vi "Do Request.vi"(7 "Processing In":refnum<class "Processing.lvclass">, 11 "TemplatedFileServe in":refnum<class "TemplatedFileServe.lvclass">) -> (0 "error out":errorcluster, 5 "Processing":refnum<class "Processing.lvclass">)   [LabVIEW 2020, in "HTTP Server.lvlib" / "TemplatedFileServe.lvclass"]
doc: "A controller's main job is to respond to a request by generating a response. The response value must be specified by calling Set Response.vi on the Processing class that's passed through the VI otherwise an error will be generated.\n\nThere are several helpers available for common response types:\nGenerating HTML content programmatically - Create Basic Response.vi\nStreaming a file from disk - Create File Response.vi\nRedirecting the user to another URL - Create Redirect Response.vi\n\nFile responses are streamed in chunks and do not load the entire file into memory at once to send in the response which allows serving large files more efficiently."
uses:
  TemplatedFileServe.lvclass
  Processing/Processing.lvclass
  Processing/Processing.lvclass/Processing.ctl
  lv-http-util/HTTP Utils/Request/Request.lvclass/Request.ctl
  lv-uri/URI/URI/URI.lvclass/URI.ctl
  TemplatedFileServe.lvclass/TemplatedFileServe.ctl
  StandardFileServe/StandardFileServe.lvclass
  lv-http-util/HTTP Utils/Request/Request.lvclass
  lv-uri/URI/URI/URI.lvclass
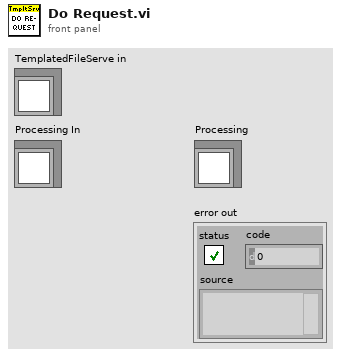
[diagram p1: front panel]
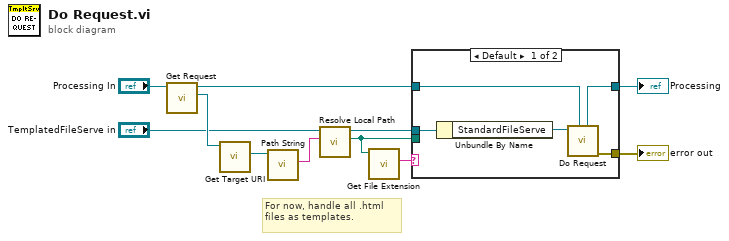
[diagram p0: block diagram]
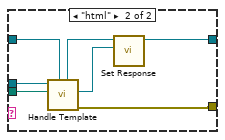
[diagram p2: hidden frame]
diagram:
  # "For now, handle all .html files as templates."
  n1 = call "Get Request.vi"("Processing in"="Processing In") -> ("Request"=w10:refnum<class "Request.lvclass">, "Processing out"=w4:refnum<class "Processing.lvclass">)  [unwired: 9 in]
  n2 = call "Get Target URI.vi"("Request in"=w10) -> ("Target URI"=w11:refnum<class "URI.lvclass">)  [unwired: 8 in, 2 out]
  n3 = call "Path String.vi"("URI in"=w11) -> ("Path String"=w7:string)  [unwired: 9 in, 1 out]
  n4 = call "Resolve Local Path.vi"("Request Path"=w7, "TemplatedFileServe in"="TemplatedFileServe in") -> ("Path"=w1:path, "TemplatedFileServe out"=w5:refnum<class "TemplatedFileServe.lvclass">)  [unwired: 7 in, 1 out]
  n5 = call <vilib>:"Get File Extension.vi"("file"=w1) -> ("lowercase file extension"=w6:string)  [unwired: 6 in, 4 out]
  n6 = case shown="Default" w6 {
    tunnel: w5 -> [w16 w22]
    tunnel: w4 -> [w14 w18]
    tunnel: [w13 w23] -> w3
    tunnel: [w12 w19] -> w2
    tunnel: w1 -> [_ w21]
    frame Default {
      n7 = Unbundle By Name(w16) -> ("StandardFileServe"=w15:refnum<class "StandardFileServe.lvclass">)
      n8 = call-dynamic "Do Request.vi"("Processing In"=w14, "StandardFileServe in"=w15) -> ("error out"=w12:errorcluster, "Processing"=w13:refnum<class "Processing.lvclass">)  [unwired: 8 in]
    }
    frame "html" {
      n9 = call "Handle Template.vi"("Processing In"=w18, "Path"=w21, "TemplatedFileServe in"=w22) -> ("error out"=w19:errorcluster, "Response"=w20:refnum<class "Response.lvclass">, "Processing"=w17:refnum<class "Processing.lvclass">)  [unwired: 5 in, 1 out]
      n10 = call "Set Response.vi"("Response"=w20, "Processing in"=w17) -> ("Processing out"=w23:refnum<class "Processing.lvclass">)  [unwired: 9 in]
    }
  }
  "error out" <- w2
  "Processing" <- w3
